vi "Enum from Value.vi"(10 "Value":i32) -> (2 "Enumeration":T1)   [LabVIEW 2020, in "ServiceType.lvlib"]
uses:
  ServiceType.lvlib
  Enumeration.ctl
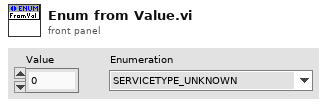
[diagram p1: front panel]
types:
  T1 = typedef "ServiceType.lvlib/Enumeration.ctl" = enum16{"SERVICETYPE_UNKNOWN", "SERVICETYPE_TCPSERVER", "SERVICETYPE_HTTPSERVER"}
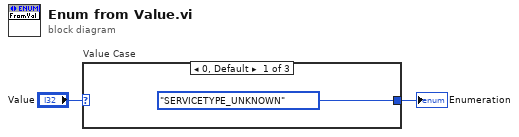
[diagram p0: block diagram]
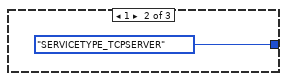
[diagram p2: hidden frame]
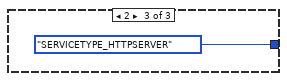
[diagram p3: hidden frame]
diagram:
  n1 = case "Value Case" shown="0, Default" "Value" {
    tunnel: [Enumeration."SERVICETYPE_UNKNOWN" ("Enumeration") Enumeration."SERVICETYPE_TCPSERVER" ("Enumeration") Enumeration."SERVICETYPE_HTTPSERVER" ("Enumeration")] -> w1
    frame 0, Default {
    }
    frame 1 {
    }
    frame 2 {
    }
  }
  "Enumeration" <- w1
